vi "GenerateConnNames.vi"(9 "Remote IP Add":string, 10 "Remote Name":string, 11 "My Name":string) -> (0 "Remote Writer":string, 1 "Remote Reader":string, 2 "My Writer":string, 3 "My Reader":string)   [LabVIEW 2020, in "NetworkConnection.lvclass"]
doc: "Generates network streams connection names based on My Name and the Remote Name.\n\nJKI Network Streams Connection 1.1.1.15\nJavier Ruiz - JKI\nCopyright (c) 2020, JKI\n\nThis library is provided \"AS IS\" ,WITHOUT WARRANTIES OR CONDITIONS OF ANY KIND, either express or implied."
uses:
  NetworkConnection.lvclass
panel:
  # "Copyright © 2020 JKI All rights reserved.\n\nAuthor: Javier Ruiz <javier.ruiz@jki.net>\n\nThis library is provided \"AS IS\" ,WITHOUT WARRANTIES OR \nCONDITIONS OF ANY KIND, either expressed or implied.\n\nJKI -- jki.net"
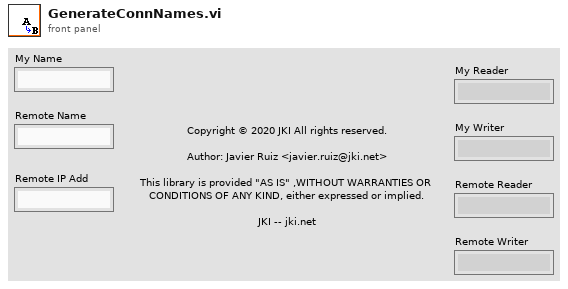
[diagram p1: front panel]
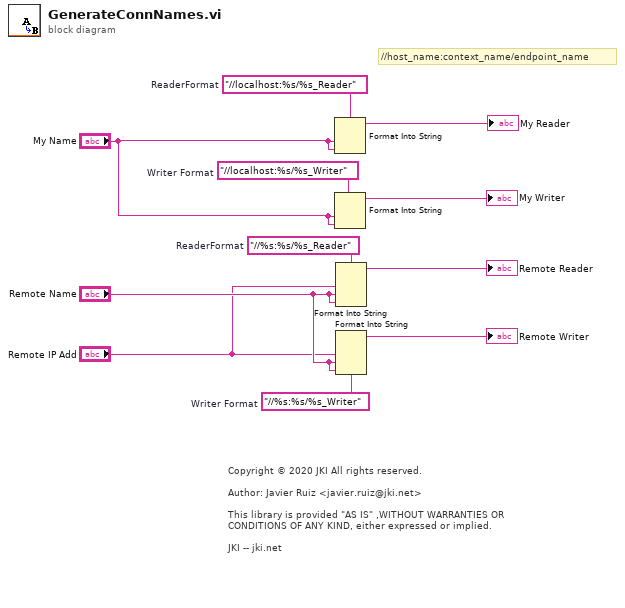
[diagram p0: block diagram]
diagram:
  w2 = "//%s:%s/%s_Reader"  # ReaderFormat
  w3 = "//%s:%s/%s_Writer"  # Writer Format
  w5 = "//localhost:%s/%s_Writer"  # Writer Format
  w6 = "//localhost:%s/%s_Reader"  # ReaderFormat
  # "//host_name:context_name/endpoint_name"
  # "Copyright © 2020 JKI All rights reserved.\n\nAuthor: Javier Ruiz <javier.ruiz@jki.net>\n\nThis library is provided \"AS IS\" ,WITHOUT WARRANTIES OR \nCONDITIONS OF ANY KIND, either expressed or implied.\n\nJKI -- jki.net"
  n1 = Format Into String(format string=w6, "My Name", "My Name") -> (resulting string=→"My Reader":string)  [unwired: 2 in, 1 out]
  n2 = Format Into String(format string=w5, "My Name", "My Name") -> (resulting string=→"My Writer":string)  [unwired: 2 in, 1 out]
  n3 = Format Into String(format string=w2, "Remote IP Add", "Remote Name", "Remote Name") -> (resulting string=→"Remote Reader":string)  [unwired: 2 in, 1 out]
  n4 = Format Into String(format string=w3, "Remote IP Add", "Remote Name", "Remote Name") -> (resulting string=→"Remote Writer":string)  [unwired: 2 in, 1 out]
